vi "DDS RAM Enable.vi"(6 "channel number (1)":u8=1 min=1 max=4 step=1, 8 "error in":errorcluster, 9 "RAM Enable":bool, 10 "RAM Dest Type":T1, 11 "DDS ref in":T2={"NI USB-8451 device reference"="", "DIO port"=0, "Serial Clock Rate [kHz]"=1000}) -> (0 "error out":errorcluster, 3 "DDS ref out":T2={"NI USB-8451 device reference"="", "DIO port"=0, "Serial Clock Rate [kHz]"=1000})   [LabVIEW 2013, in "DDS.lvlib"]
doc: "This VI will enable or disable the RAM bit as appropriate and also programs the correct values into the RAM destination bits."
uses:
  DDS.lvlib
  Controls/DDS Box Device Reference.ctl
  <vilib>/ni845x/ni845x.llb/ni845xControl.ctl
  Controls/DDS RAM Destination.ctl
  Controls/AD9910 registers.ctl
panel:
  out "CFR1":u8[](array[numeric])
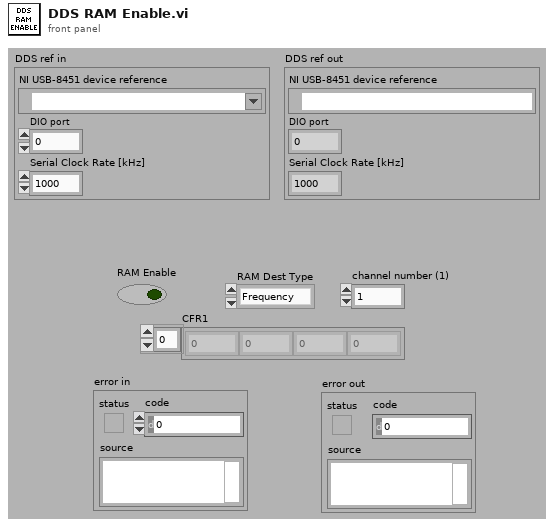
[diagram p1: front panel]
types:
  T1 = typedef "DDS.lvlib/DDS RAM Destination.ctl" = enum16{"Frequency", "Phase", "Amplitude", "Polar"}
  T2 = typedef "DDS.lvlib/DDS Box Device Reference.ctl" = cluster{"NI USB-8451 device reference":T3, "DIO port":u8, "Serial Clock Rate [kHz]":u16}
  T3 = typedef "ni845xControl.ctl" = refnum<k21>
  T4 = typedef "DDS.lvlib/AD9910 registers.ctl" = enum16{"CFR1", "CFR2", "CFR3", "Auxiliary DAC Control", "I/0 Update Rate", "Frequency Tuning Word", "Phase Offset Word", "Amplitude Scale Factor", "Multichip Sync", "Digital Ramp Limit", "Digital Ramp Step Size", "Digital Ramp Rate", "Single Tone Profile 0", "Single Tone Profile 1", "Single Tone Profile 2", "Single Tone Profile 3", "Single Tone Profile 4", "Single Tone Profile 5", "Single Tone Profile 6", "Single Tone Profile 7", "RAM Profile 0", "RAM Profile 1", "RAM Profile 2", "RAM Profile 3", "RAM Profile 4", "RAM Profile 5", "RAM Profile 6", "RAM Profile 7", "RAM"}
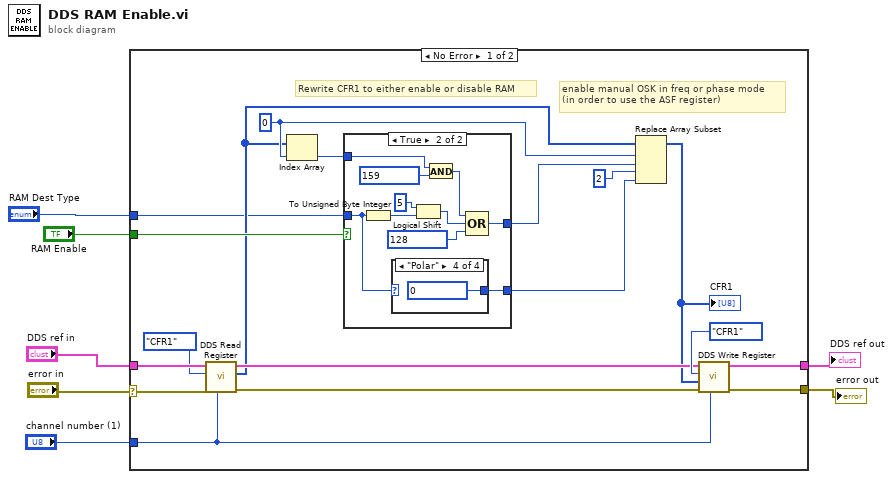
[diagram p0: block diagram]
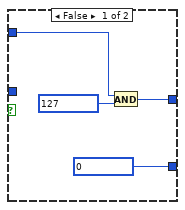
[diagram p2: hidden frame]
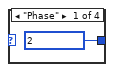
[diagram p3: hidden frame]
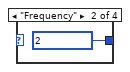
[diagram p4: hidden frame]
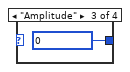
[diagram p5: hidden frame]
diagram:
  n1 = case shown="No Error" "error in" {
    selector: "error in" -> [w12 w45]
    tunnel: [w25 w44] -> w5
    tunnel: [w24 w45] -> w6
    tunnel: "DDS ref in" -> [w22 w44]
    tunnel: "channel number (1)" -> [w18 _]
    tunnel: "RAM Enable" -> [w11 _]
    tunnel: "RAM Dest Type" -> [w9 _]
    frame No Error {
      w14 = 0 ("index")
      # "enable manual OSK in freq or phase mode\n(in order to use the ASF register)"
      # "Rewrite CFR1 to either enable or disable RAM"
      n2 = call "DDS Read Register.vi"("channel number (1)"=w18, "error in (no error)"=w12, "Register"=AD9910_registers."CFR1", "DDS ref in"=w22) -> ("error out"=w21:errorcluster, "Read data"=w10:u8[], "DDS ref out"=w20:T2)  [unwired: 5 in]
      n3 = Index Array(array=w10, index=w14) -> (element=w13:u8)
      n4 = case shown="True" w11 {
        tunnel: w9 -> [_ w30]
        tunnel: w13 -> [w28 w32]
        tunnel: [w27 w38] -> w15
        tunnel: [u8 0 ("new element/subarray") w31] -> w17
        frame False {
          n5 = And(x=w28, y=u8 127) -> (x .and. y?=w27:u8)
        }
        frame True {
          n6 = To Unsigned Byte Integer(number=w30) -> (unsigned 8bit integer=w37:u8)
          n7 = case shown="\"Polar\"" w30 {
            tunnel: [u8 2 ("new element/subarray") u8 2 ("new element/subarray") u8 0 ("new element/subarray") u8 0 ("new element/subarray")] -> w31
            frame "Phase" {
            }
            frame "Frequency" {
            }
            frame "Amplitude" {
            }
            frame "Polar" {
            }
          }
          n8 = Logical Shift(y=i8 5, x=w37) -> (x << y=w35:u8)
          n9 = And(x=w32, y=u8 159) -> (x .and. y?=w33:u8)
          n10 = Compound Arithmetic op=OR(w33, w35, u8 128 ("y")) -> (w38:u8)
        }
      }
      n11 = Replace Array Subset(array=w10, new element #1=w15, index #1=w14, new element #2=w17, index #2=2 ("index")) -> (w8:u8[])
      "CFR1" <- w8
      n12 = call "DDS Write Register.vi"("channel number (1)"=w18, "error in (no error)"=w21, "Write Data"=w8, "Register"=AD9910_registers."CFR1", "DDS ref in"=w20) -> ("error out"=w24:errorcluster, "DDS ref out"=w25:T2)  [unwired: 4 in, 1 out]
    }
    frame Error {
    }
  }
  "error out" <- w6
  "DDS ref out" <- w5
